vi "PH_BeamlineInformation.set GUI elements to default.vi"(0 "i ref in":refnum<vi>, 5 "error in (no error)":errorcluster) -> (14 "i ref out":refnum<vi>, 19 "error out":errorcluster)   [LabVIEW 2014, in "PH_BeamlineInformation.lvlib"]
doc: "This VI sets some GUI elements to dafault (start) values."
uses:
  PH_BeamlineInformation.lvlib
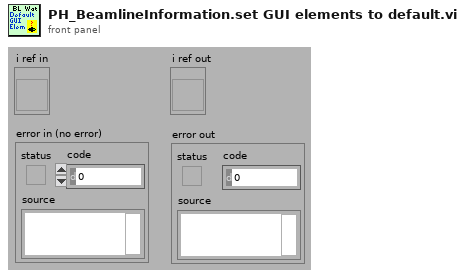
[diagram p1: front panel]
types:
  T1 = typedef "PH_BeamlineInformation.lvlib/PH_BeamlineInformation.i attribute.ctl" = cluster{"BL GUI Elements of Services":cluster{"Service Name":string, "GUI Elements":refnum<vi>[], "Status":i32}[], "Powermeters":T2, "Efficiency":T3, "Heads":T4[]}
  T2 = typedef "PH_BeamlineInformation.lvlib/PH_BeamlineInformation.Powermeter.ctl" = cluster{"ns FE":cluster{"GUI Ref":refnum<vi>, "Value":dbl}, "fs FE":cluster{"GUI Ref":refnum<vi>, "Value":dbl}, "PA":cluster{"GUI Ref":refnum<vi>, "Value":dbl}, "MA":cluster{"GUI Ref":refnum<vi>, "Value":dbl}, "Z6 green":cluster{"GUI Ref":refnum<vi>, "Value":dbl}, "Z6 IR":cluster{"GUI Ref":refnum<vi>, "Value":dbl}, "Z6 COS":cluster{"GUI Ref":refnum<vi>, "Value":dbl}}
  T3 = typedef "PH_BeamlineInformation.lvlib/PH_BeamlineInformation.Efficiency.ctl" = cluster{"PA Gain":cluster{"GUI Ref":refnum<vi>, "Value":dbl}, "MA Gain":cluster{"GUI Ref":refnum<vi>, "Value":dbl}, "Z6 green Conversion":cluster{"GUI Ref":refnum<vi>, "Value":dbl}, "Z6 Comp Losses":cluster{"GUI Ref":refnum<vi>, "Value":dbl}}
  T4 = typedef "PH_BeamlineInformation.lvlib/PH_BeamlineInformation.Head.ctl" = cluster{"PowerUnit":T5, "in use":cluster{"Value":bool, "GUI Ref":refnum<vi>, "linked":bool}, "voltage":cluster{"Value":dbl, "GUI Ref":refnum<vi>, "linked":bool}}
  T5 = typedef "PH_PP_Common.lvlib/PH_PP_Common.PUs.ctl" = enum16{"no Info", "PA-19mm-1", "PA-19mm-2", "PA-45mm-PILC", "PA-45mm-MAIN", "MA-PU-1", "MA-PU-2", "MA-PU-3", "MA-PU-4", "MA-PU-5", "MA-PU-6", "MA-FR", "MA-PILC", "PA-45mm-DP"}
  T6 = cluster{"Service Name":string, "GUI Elements":refnum<vi>[], "Status":i32}[]
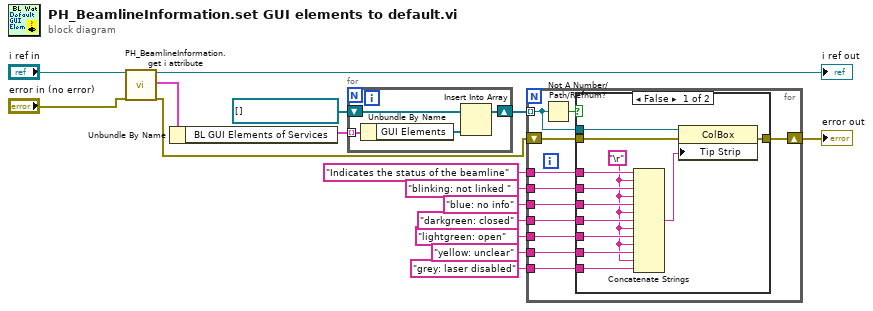
[diagram p0: block diagram]
diagram:
  n1 = call "PH_BeamlineInformation.get i attribute.vi"("i ref in"="i ref in", "error in (no error)"="error in (no error)") -> ("i ref out"=→"i ref out":refnum<vi>, "i attribute"=w14:T1, "error out"=w1:errorcluster)  [unwired: 15 in]
  n2 = Unbundle By Name(w14) -> ("BL GUI Elements of Services"=w3:T6)
  n3 = for {
    shift-right: [w18] -> w2
    shift-left: refnum<vi>[] [] -> [w17]
    tunnel: w3 -> [w20] mode=indexing
    n4 = Unbundle By Name(w20) -> ("GUI Elements"=w19:refnum<vi>[])
    n5 = Insert Into Array(array=w17, new element=w19) -> (w18:refnum<vi>[])  [unwired: 1 in]
  }
  n6 = for {
    tunnel: "blinking: not linked " ("string") -> [w31]
    tunnel: "blue: no info" ("string") -> [w30]
    shift-right: [w29] -> w10
    shift-left: w1 -> [w28]
    tunnel: "Indicates the status of the beamline" ("string") -> [w26]
    tunnel: w2 -> [w21] mode=indexing
    tunnel: "darkgreen: closed" ("string") -> [w25]
    tunnel: "lightgreen: open" ("string") -> [w24]
    tunnel: "yellow: unclear" ("string") -> [w23]
    tunnel: "grey: laser disabled" ("string") -> [w22]
    n7 = Not A Number/Path/Refnum?(number/path/refnum=w21) -> (NaN/Path/Refnum?=w27:bool)
    n8 = case shown="False" w27 {
      tunnel: w31 -> [w42 _]
      tunnel: w30 -> [w41 _]
      tunnel: [w40 w44] -> w29
      tunnel: w28 -> [w37 w44]
      tunnel: w26 -> [w39 _]
      tunnel: w21 -> [w38 _]
      tunnel: w25 -> [w36 _]
      tunnel: w24 -> [w35 _]
      tunnel: w23 -> [w34 _]
      tunnel: w22 -> [w33 _]
      frame False {
        w32 = "\r"
        n9 = Concatenate Strings(w39, w32, w42, w32, w41, w32, w36, w32, w35, w32, w34, w32, w33) -> (w43:string)
        n10 = property class="ColBox"(reference=w38, error in=w37, "Tip Strip"=w43) -> (error out=w40:errorcluster)  [unwired: 1 out]
      }
      frame True {
      }
    }
  }
  "error out" <- w10
